vi "OAT Factor Decomposition.vi"(7 "number":i32) -> (0 "error":bool, 1 "counts":i32[](array[numeric]), 2 "different factors":i32[](array[numeric]), 3 "factors":i32[](array[numeric]))   [LabVIEW 2017, in "SoundVib_Resampling.lvlib"]
uses:
  <vilib>/addons/Sound and Vibration/Order Analysis/Resample Order Tracking/SoundVib_Resampling.lvlib
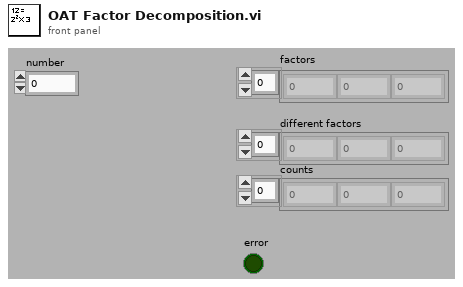
[diagram p1: front panel]
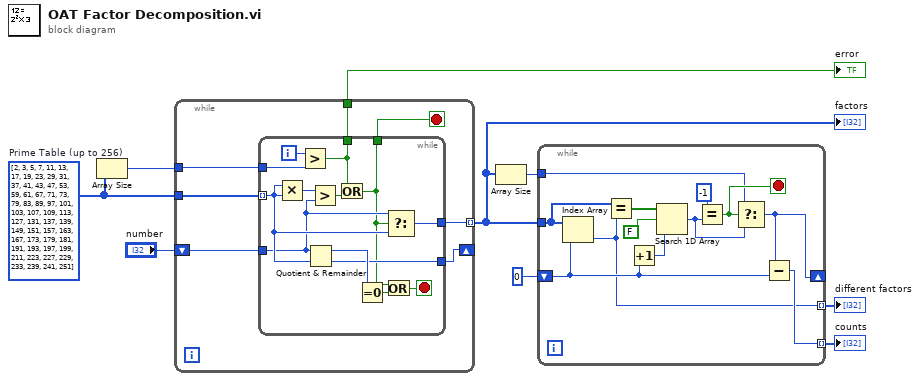
[diagram p0: block diagram]
diagram:
  w1 = i32[] [2, 3, 5, 7, 11, 13, 17, 19, 23, 29, 31, 37, 41, 43, 47, 53, 59, 61, 67, 71, 73, 79, 83, 89, 97, 101, 103, 107, 109, 113, 127, 131, 137, 139, 149, 151, 157, 163, 167, 173, 179, 181, 191, 193, 197, 199, 211, 223, 227, 229, 233, 239, 241, 251]  # Prime Table (up to 256)
  n1 = Array Size(array=w1) -> (size(s)=w9:i32)
  n2 = while {
    tunnel: [w11] -> w7
    tunnel: [w13] -> w2 mode=indexing
    shift-left: "number" -> [w14]
    shift-right: [w10] -> _
    tunnel: w9 -> [w15]
    tunnel: w1 -> [w16]
    stop <- w12 stop-if-true
    n3 = while {
      tunnel: [w17] -> w11
      tunnel: [w21] -> w12
      tunnel: [w27] -> w13
      tunnel: [w28] -> w10
      tunnel: w14 -> [w24]
      tunnel: w15 -> [w19]
      tunnel: w16 -> [w26] mode=indexing
      i -> [w20]
      stop <- w22 stop-if-true
      n4 = Multiply(x=w26, y=w26) -> (x*y=w25:i32)
      n5 = Greater?(x=w20, y=w19) -> (0:w17:bool)
      n6 = Quotient & Remainder(x=w24, y=w26) -> (x-y*floor(x/y)=w29:i32, floor(x/y)=w28:i32)
      n7 = Greater?(x=w25, y=w24) -> (0:w18:bool)
      n8 = Or(x=w17, y=w18) -> (x .or. y?=w21:bool)
      n9 = Equal To 0?(x=w29) -> (x = 0?=w23:bool)
      n10 = Or(x=w21, y=w23) -> (x .or. y?=w22:bool)
      n11 = Select(t=w24, s=w21, f=w26) -> (s? t:f=w27:i32)
    }
  }
  "factors" <- w2
  "error" <- w7
  n12 = Array Size(array=w2) -> (size(s)=w5:i32)
  n13 = while {
    tunnel: [w30] -> w4 mode=indexing
    tunnel: [w31] -> w3 mode=indexing
    tunnel: w5 -> [w34]
    shift-left: 0 -> [w32]
    shift-right: [w33] -> _
    tunnel: w2 -> [w41]
    stop <- w37 stop-if-true
    n14 = Index Array(array=w41, index=w32) -> (element=w30:i32)
    n15 = Equal?(x=w41, y=w30) -> (x = y?=w40:bool[])
    n16 = Increment(x=w32) -> (x+1=w38:i32)
    n17 = Search 1D Array(1D array=w40, element=FALSE, start index (0)=w38) -> (index of element=w35:i32)
    n18 = Equal?(x=-1 ("y"), y=w35) -> (x = y?=w37:bool)
    n19 = Select(t=w34, s=w37, f=w35) -> (s? t:f=w33:i32)
    n20 = Subtract(x=w33, y=w32) -> (x-y=w31:i32)
  }
  "different factors" <- w4
  "counts" <- w3
